vi "Test Process Multiple Start.vi"(8 "error in (no error)":errorcluster, 11 "Process Test In":refnum<class "Process Dev Test.lvclass">) -> (0 "error out":errorcluster, 3 "Process Test Out":refnum<class "Process Dev Test.lvclass">)   [LabVIEW 2020, in "Process Dev Test.lvclass"]
uses:
  Process Dev Test.lvclass
  C:/Program Files (x86)/National Instruments/LabVIEW 2020/vi.lib/Astemes/LUnit/Test Case.lvclass
  source/Framework Test Suite/Mock Error Handler/Mock Error Handler.lvclass
  C:/Git/astemes-triarc-framework/source/Framework/Error Handler Interface/Error Handler Interface.lvclass
  source/Framework/Process/Process.lvclass/Process.ctl
  <vilib>/Astemes/LUnit/Test Case.lvclass/Test Case.ctl
  <vilib>/Astemes/LUnit/LUnit Assertion Result.lvclass/LUnit Assertion Result.ctl
  <vilib>/Astemes/LUnit/LUnit Test Case Result.lvclass/LUnit Test Case Result.ctl
  <vilib>/Astemes/LUnit/LUnit Method Result.lvclass/LUnit Method Result.ctl
  source/Framework/Process/Protected/Messaging/Enqueue Message.vi
  source/Framework/Process/Public/Lifecycle/Get Lifecycle State.vi
  <vilib>/Astemes/LUnit/Palette/Pass.vi
  <vilib>/Astemes/LUnit/Palette/Fail.vi
  <vilib>/Astemes/LUnit/Set Assertion Type.vi
  source/Framework/Process/Private/SubVIs/Wait for finish.vi
  source/Framework/Process/Private/SubVIs/Set Lifecycle State.vi
  source/Framework/Process/Private/SubVIs/Handle Debug Data.vi
  <vilib>/Utility/error.llb/Clear Errors.vi
  <vilib>/Astemes/LUnit/Add test result.vi
  <vilib>/Astemes/LUnit/LUnit Write Passed.vi
  <vilib>/Astemes/LUnit/LUnit Write Message.vi
  <vilib>/Astemes/LUnit/LUnit Write Description.vi
  <vilib>/Astemes/LUnit/LUnit Write Assertion Type.vi
  source/Framework/Logging/Log Debug.vi
  <vilib>/AdvancedString/1D String Array to Delimited String.vi
  <vilib>/Utility/High Resolution Relative Seconds.vi
  <vilib>/Astemes/LUnit/LUnit Record Assertion Result.vi
  <vilib>/Astemes/LUnit/LUnit Aggregate Assertion Results.vi
  <vilib>/Astemes/LUnit/Assertion Result/LUnit Read Status.vi
  <vilib>/Astemes/LUnit/LUnit Read Message.vi
  <vilib>/Astemes/LUnit/LUnit Read Description.vi
  <vilib>/Astemes/LUnit/Method Result/LUnit Merge Status.vi
  <vilib>/Astemes/LUnit/LUnit Concatenate result strings.vi
  <vilib>/Utility/error.llb/Error Cluster From Error Code.vi
  source/Framework/Process/Public/Read Name.vi
  <vilib>/Astemes/LUnit/LUnit Assertion Result.lvclass
  source/Framework/Process/Process.lvclass
  <vilib>/Astemes/LUnit/Test Case.lvclass
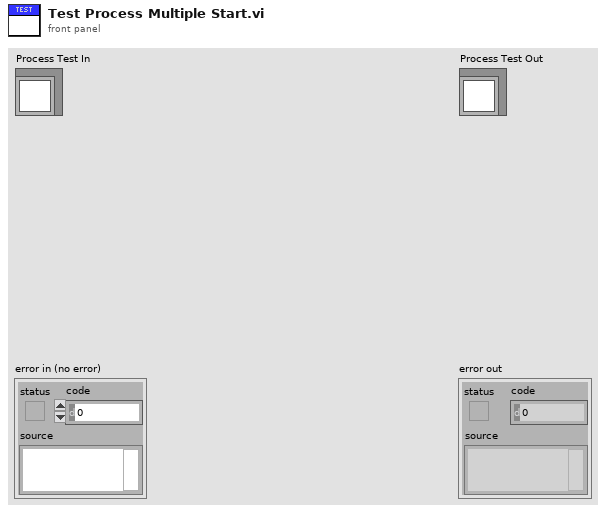
[diagram p1: front panel]
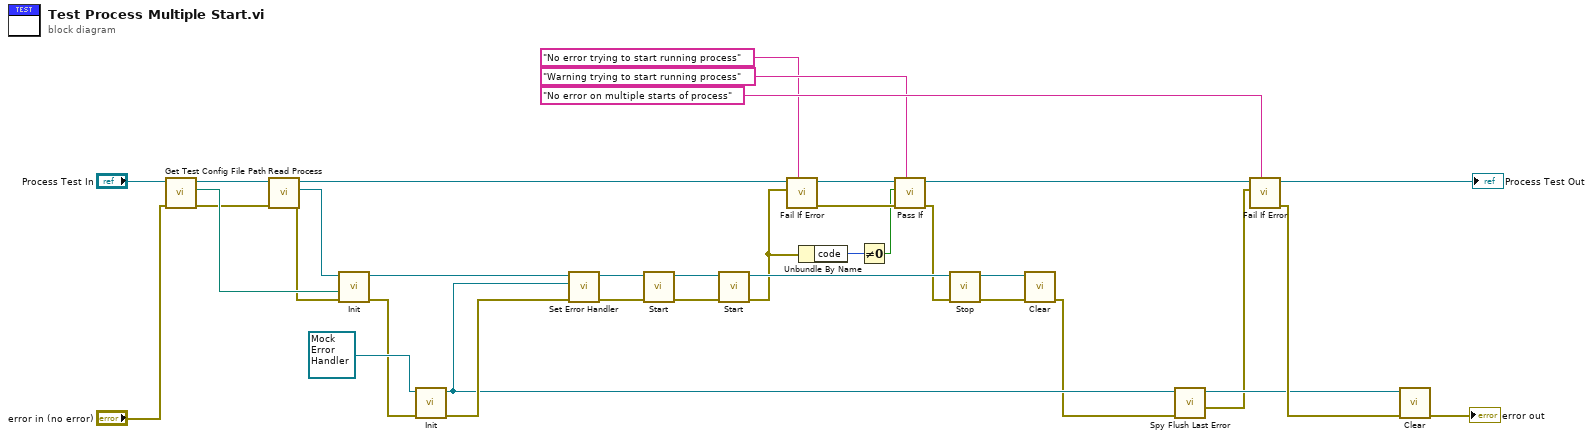
[diagram p0: block diagram]
diagram:
  n1 = call "Get Test Config File Path.vi"("error in (no error)"="error in (no error)", "Process Test In"="Process Test In") -> ("error out"=w27:errorcluster, "Test config path"=w30:path, "Process Test Out"=w32:refnum<class "Process Dev Test.lvclass">)  [unwired: 7 in]
  n2 = call "Read Process.vi"("error in (no error)"=w27, "Process Test in"=w32) -> ("error out"=w28:errorcluster, "Process.lvclass"=w29:refnum<class "Process.lvclass">, "Process Test out"=w5:refnum<class "Process Dev Test.lvclass">)  [unwired: 7 in]
  n3 = call-dynamic "Init.vi"("error in (no error)"=w28, "Config File Path"=w30, "Process In"=w29) -> ("error out"=w17:errorcluster, "Process Out"=w33:refnum<class "Process.lvclass">)  [unwired: 7 in]
  n4 = call-dynamic "Init.vi"("error in (no error)"=w17, "Mock Error Handler In"=refnum<class "Mock Error Handler.lvclass"> refnum ("Mock Error Handler.lvclass")) -> ("error out"=w21:errorcluster, "Mock Error Handler Out"=w20:refnum<class "Mock Error Handler.lvclass">)  [unwired: 8 in]
  n5 = call "Set Error Handler.vi"("error in (no error)"=w21, "Error Handler"=w20, "Process In"=w33) -> ("error out"=w22:errorcluster, "Process Out"=w23:refnum<class "Process.lvclass">)  [unwired: 7 in]
  n6 = call "Start.vi"("error in (no error)"=w22, "Process In"=w23) -> ("error out"=w35:errorcluster, "Process Out"=w36:refnum<class "Process.lvclass">)  [unwired: 7 in, 1 out]
  n7 = call "Start.vi"("error in (no error)"=w35, "Process In"=w36) -> ("error out"=w4:errorcluster, "Process Out"=w26:refnum<class "Process.lvclass">)  [unwired: 7 in, 1 out]
  n8 = call <vilib>:"Fail If Error.vi"("Description"="No error trying to start running process", "Assert error"=w4, "LUnit Test Case In"=w5) -> ("error out"=w10:errorcluster, "LUnit Test Case Out"=w11:refnum<class "Process Dev Test.lvclass">)  [unwired: 7 in]
  n9 = Unbundle By Name(w4) -> ("code"=w9:i32)
  n10 = Not Equal To 0?(x=w9) -> (x != 0?=w8:bool)
  n11 = call <vilib>:"Pass If.vi"("Description"="Warning trying to start running process", "error in (no error)"=w10, "Pass?"=w8, "LUnit Test Case In"=w11) -> ("error out"=w3:errorcluster, "LUnit Test Case Out"=w2:refnum<class "Process Dev Test.lvclass">)  [unwired: 6 in]
  n12 = call "Stop.vi"("error in (no error)"=w3, "Process In"=w26) -> ("error out"=w24:errorcluster, "Process Out"=w25:refnum<class "Process.lvclass">)  [unwired: 7 in, 1 out]
  n13 = call-dynamic "Clear.vi"("error in (no error)"=w24, "Process In"=w25) -> ("error out"=w16:errorcluster)  [unwired: 9 in]
  n14 = call "Spy Flush Last Error.vi"("error in (no error)"=w16, "Mock Error Handler In"=w20) -> ("Error"=w1:errorcluster, "Mock Error Handler Out"=w14:refnum<class "Mock Error Handler.lvclass">)  [unwired: 7 in, 1 out]
  n15 = call <vilib>:"Fail If Error.vi"("Description"="No error on multiple starts of process", "Assert error"=w1, "LUnit Test Case In"=w2) -> ("error out"=w15:errorcluster, "LUnit Test Case Out"=→"Process Test Out":refnum<class "Process Dev Test.lvclass">)  [unwired: 7 in]
  n16 = call-dynamic "Clear.vi"("error in (no error)"=w15, "Mock Process In"=w14) -> ("error out"=→"error out":errorcluster)  [unwired: 9 in]
